vi "Write AllowUndefinedNames.vi"(5 "Allow Undefined Names":bool, 9 "VisaResourceName in":refnum<class "VisaResourceName.lvclass">) -> (3 "VisaResourceName out":refnum<class "VisaResourceName.lvclass">)   [LabVIEW 2014, in "Raspberry Pi Compatible Compiler for LabVIEW.lvlib" / "VisaResourceName.lvclass"]
uses:
  VisaResourceName.lvclass
  VisaResourceName.lvclass/VisaResourceName.ctl
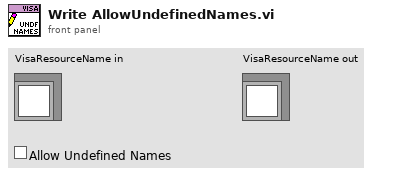
[diagram p1: front panel]
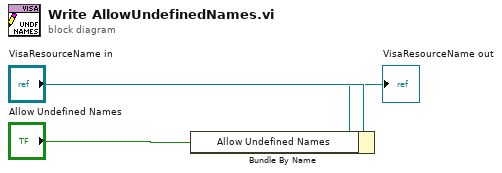
[diagram p0: block diagram]
diagram:
  n1 = Bundle By Name(cluster="VisaResourceName in", "Allow Undefined Names"="Allow Undefined Names") -> (→"VisaResourceName out":refnum<class "VisaResourceName.lvclass">)
